vi "LoadAll.vi"   [LabVIEW 2022 SP3]
uses:
  Classes/DAQWFE/LV_Source/Subsystems/DAQ/DAQ.lvclass
  <vilib>/Analysis/NI_AALPro.lvlib
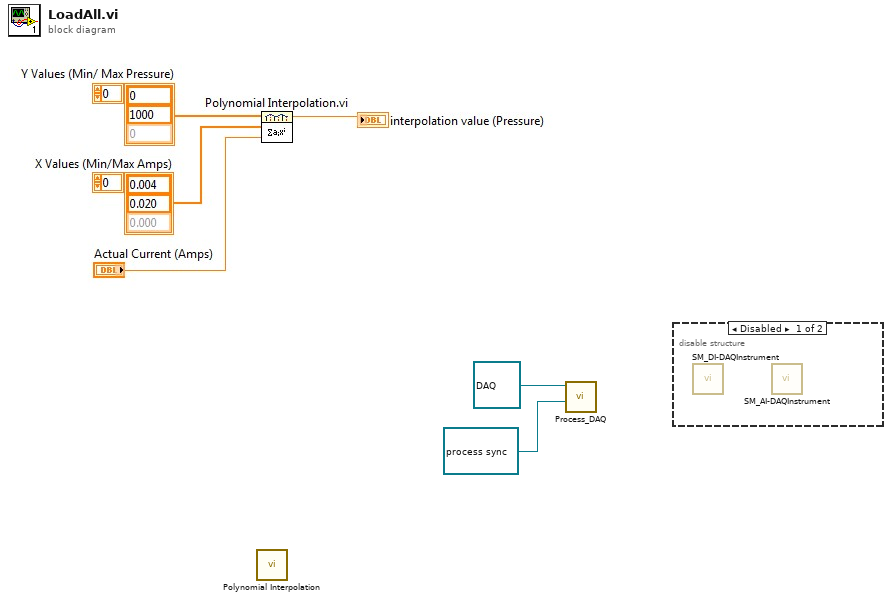
[diagram p0: block diagram]
diagram:
  n1 = call <vilib>:"Polynomial Interpolation.vi"() -> ()  [unwired: 3 in, 3 out]
  n2 = call "Process_DAQ.vi"("start process sync notifier"=refnum<notifier> refnum, "DAQ"=refnum<class "DAQ.lvclass"> refnum) -> ()  [unwired: 9 in, 1 out]
  n3 = disable-structure shown="Disabled" {
    frame Disabled {
      n4 = call "SM_DI-DAQInstrument.vi"() -> ()  [unwired: 11 in, 1 out]
      n5 = call "SM_AI-DAQInstrument.vi"() -> ()  [unwired: 11 in, 1 out]
    }
    frame Enabled {
    }
  }
